vi "ReversedEngineering GetInheritanceClasses.vi"(1 "classInfos":T1[](array[typedef]), 2 "classPath":path) -> (15 "baseClasses":path[](array[path]))   [LabVIEW 2012]
uses:
  <resource>/Framework/Providers/Open_GDS/UML/ReversedEngineering/ReversedEngineering ClassInfoType.ctl
  <resource>/Framework/Providers/Open_GDS/UML/UMLEditor/UMLEditor_VisibilityType.ctl
  <resource>/Framework/Providers/Open_GDS/UML/ReversedEngineering/ReversedEngineering AttributeInfoType.ctl
  <resource>/Framework/Providers/Open_GDS/UML/ReversedEngineering/ReversedEngineering AttributeDataType.ctl
  <resource>/Framework/Providers/Open_GDS/UML/ReversedEngineering/ReversedEngineering_ClassDependencyDetailsType.ctl
  <resource>/Framework/Providers/Open_GDS/ClassProviders/Common/ScriptingFunctions/SubVIs/Scripting_ViDependencyType.ctl
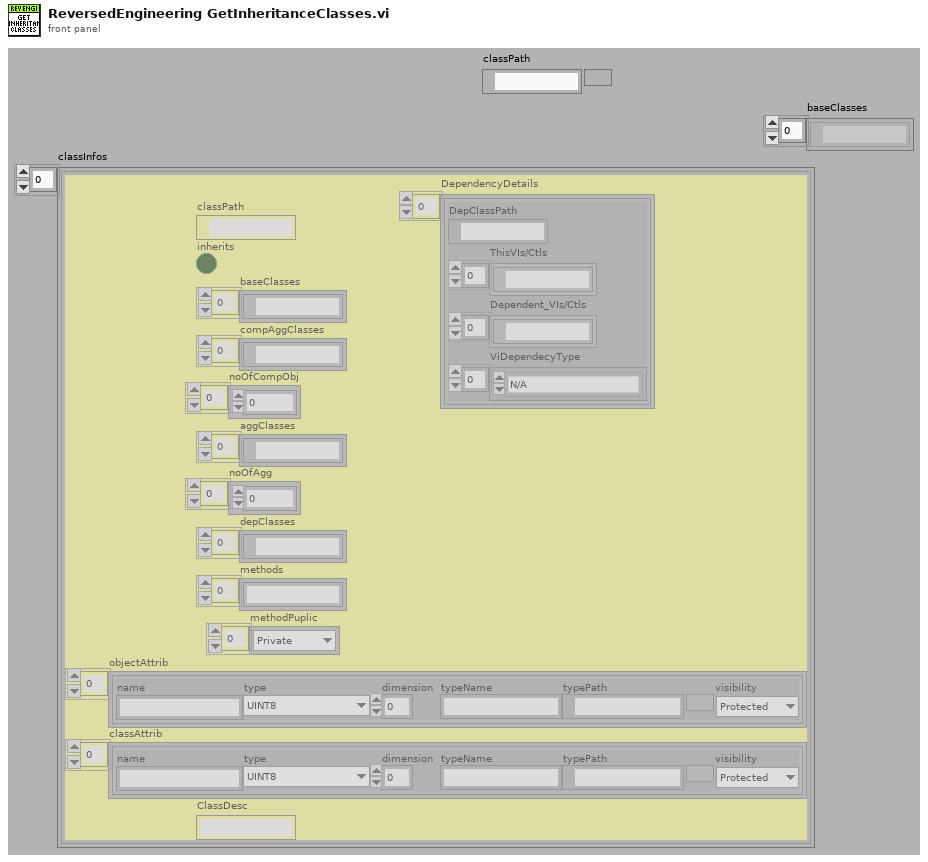
[diagram p1: front panel]
types:
  T1 = typedef "ReversedEngineering ClassInfoType.ctl" = cluster{"classPath":path, "inherits":bool, "baseClasses":path[], "compAggClasses":path[], "noOfCompObj":i32[], "aggClasses":path[], "noOfAgg":i32[], "depClasses":path[], "methods":string[], "methodPuplic":T2[], "objectAttrib":T3[], "classAttrib":T3[], "ClassDesc":string, "DependencyDetails":T5[]}
  T2 = typedef "UMLEditor_VisibilityType.ctl" = enum16{"Public", "Private", "Protected"}
  T3 = typedef "ReversedEngineering AttributeInfoType.ctl" = cluster{"name":string, "type":T4, "dimension":i32, "typeName":string, "typePath":path, "visibility":T2}
  T4 = typedef "ReversedEngineering AttributeDataType.ctl" = enum16{"UINT8", "INT8", "UINT16", "INT16", "UINT32", "INT32", "UINT64", "INT64", "SGL", "DBL", "EXT", "CSG", "CDB", "CXT", "TimeStamp", "STRING", "PATH", "BOOL", "ENUM", "RefNum", "VIRefNum", "ClassRefNum", "Cluster", "Variant", "TypeRef", "Waveform", "LabVIEW Object", "Other"}
  T5 = typedef "ReversedEngineering_ClassDependencyDetailsType.ctl" = cluster{"DepClassPath":path, "ThisVIs/Ctls":path[], "Dependent_VIs/Ctls":path[], "ViDependecyType":T6[]}
  T6 = typedef "Scripting_ViDependencyType.ctl" = enum16{"N/A", "Launches"}
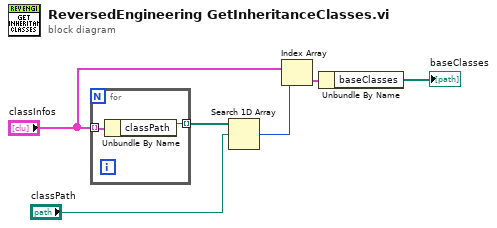
[diagram p0: block diagram]
diagram:
  n1 = for {
    tunnel: "classInfos" -> [w8] mode=indexing
    tunnel: [w7] -> w5 mode=indexing
    n2 = Unbundle By Name(w8) -> ("classPath"=w7:path)
  }
  n3 = Search 1D Array(1D array=w5, element="classPath") -> (index of element=w4:i32)  [unwired: 1 out]
  n4 = Index Array(array="classInfos", index=w4) -> (element=w3:T1)
  n5 = Unbundle By Name(w3) -> ("baseClasses"=→"baseClasses":path[])
